vi "Feedback Node - Enable Terminal.vi"() -> ()   [LabVIEW 2023]
doc: "Demonstrates the use of the Enable Terminal to control the execution of a Feedback Node. When the value of the Enable Terminal is TRUE, the Feedback Node functions normally. When the value of the Enable Terminal is FALSE, the Feedback Node ignores the current input value and retains its stored value for the next iteration."
panel:
  out "Random Data (Shift Register)":dbl[](graph)
  out "Random Data (Feedback Node)":dbl[](graph)
  in  "Upper Limit":dbl(slide)=0.5 scale=0.0..1.0
  in  "Stop":bool
  # "Overview: Demonstrates the use of the Enable Terminal to control the execution of a Feedback Node.\nInstructions:\nRun the VI. It will display data accumulated across all iterations of a loop, but only if that data is lower than the Upper Limit value. See the block diagram for more information."
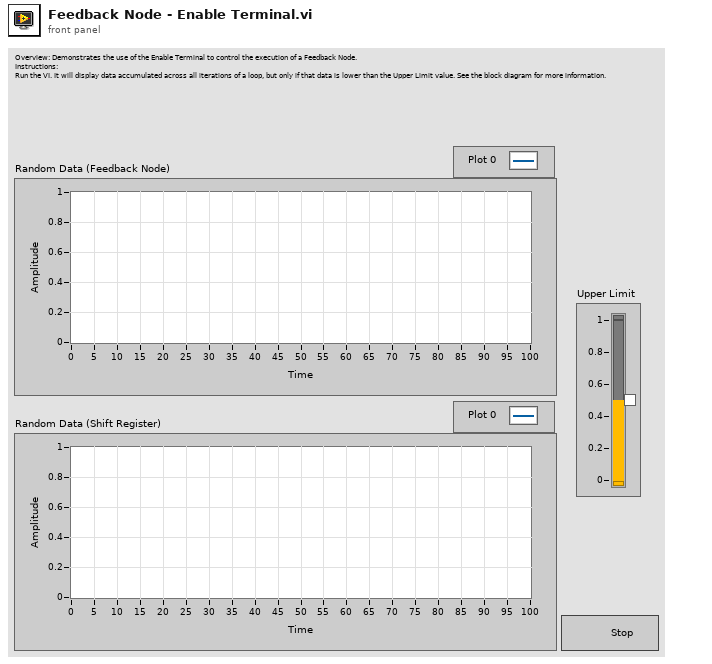
[diagram p1: front panel]
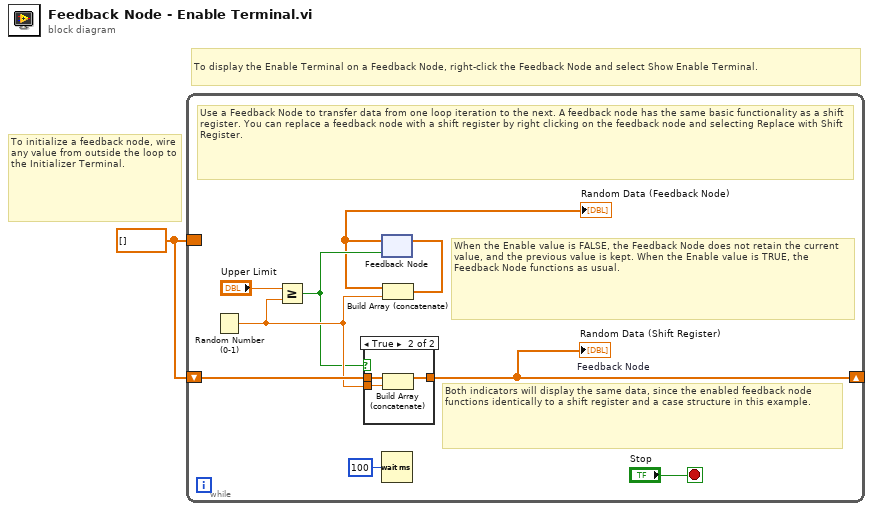
[diagram p0: block diagram]
diagram:
  w1 = dbl[] []
  # "To display the Enable Terminal on a Feedback Node, right-click the Feedback Node and select Show Enable Terminal."
  # "To initialize a feedback node, wire any value from outside the loop to the Initializer Terminal."
  n1 = while {
    border: w1 -> [_]
    shift-right: [w7] -> _
    shift-left: w1 -> [w9]
    stop <- "Stop" stop-if-true
    # "When the Enable value is FALSE, the Feedback Node does not retain the current value, and the previous value is kept. When the Enable value is TRUE, the Feedback Node functions as usual."
    # "Both indicators will display the same data, since the enabled feedback node functions identically to a shift register and a case structure in this example."
    # "Use a Feedback Node to transfer data from one loop iteration to the next. A feedback node has the same basic functionality as a shift register. You can replace a feedback node with a shift register by right clicking on the feedback node and selecting Replace with Shift Register."
    n2 = Random Number (0-1)() -> (number: 0 to 1=w4:dbl)
    n3 = Greater Or Equal?(x="Upper Limit", y=w4) -> (x >= y?=w3:bool)
    n4 = case shown="True" w3 {
      tunnel: w9 -> [w11 w14]
      tunnel: [w11 w13] -> w7
      tunnel: w4 -> [_ w12]
      frame False {
      }
      frame True {
        n5 = Build Array (concatenate)(w14, w12) -> (w13:dbl[])
      }
    }
    "Random Data (Shift Register)" <- w7
    n6 = feedback #1 "Feedback Node"() -> (w2:dbl[])
    "Random Data (Feedback Node)" <- w2
    n7 = Wait (ms)(milliseconds to wait=u32 100) -> ()  [unwired: 1 out]
    n8 = Build Array (concatenate)(w2, w4) -> (w8:dbl[])
    n9 = feedback-in #1(w8, w3) -> ()
  }
